vi "TestMath.vi"() -> ()   [LabVIEW 2016]
panel:
  in  "Limits":cluster{dbl, dbl}(slide)={0.0, 0.24242424242424243} scale=0.0..1.0
  out "Yout from machine":dbl
  out "Xout from machine":dbl
  in  "Yin":dbl
  in  "Xin":dbl
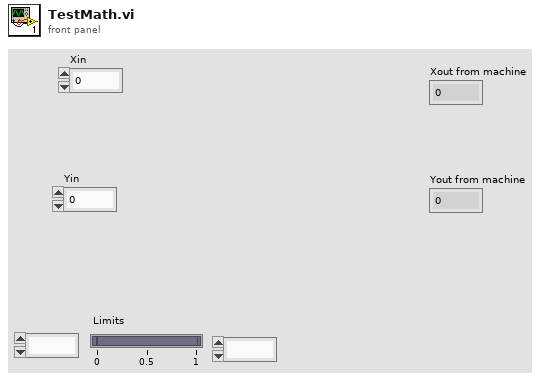
[diagram p1: front panel]
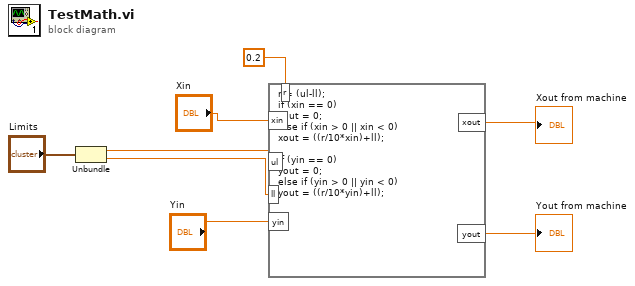
[diagram p0: block diagram]
diagram:
  n1 = Unbundle("Limits") -> (w2:dbl, w1:dbl)
  n2 = formula code="r = (ul-ll);\nif (xin == 0)\nxout = 0;\nelse if (xin > 0 || xin < 0)\nxout = ((r/10*xin)+ll);\n\nif (yin == 0)\nyout = 0;\nelse if (yin > 0 || yin < 0)\nyout = ((r/10*yin)+ll);"("xin"="Xin", "yin"="Yin", "ul"=w2, "ll"=w1, "r"=0.2 ("input variable")) -> ("xout"=→"Xout from machine":dbl, "yout"=→"Yout from machine":dbl)
